vi "Noise Generation.vi"() -> ()   [LabVIEW 2019]
doc: "Generates a monotone signal. If you are setting up a demo system of active noise control, you can use this VI to simulate a noisy environment with monotone noise."
uses:
  <vilib>/sound2/lvsound2.llb/Sampling Mode.ctl
  <vilib>/sound2/lvsound2.llb/Sound Data Format.ctl
  <vilib>/sound2/lvsound2.llb/Sound Output Set Volume (Single).vi
  <vilib>/sound2/lvsound2.llb/Sound Output Write (DBL).vi
  <vilib>/measure/NI_MABase.lvlib
panel:
  in  "Amplitude":dbl(slide)=1.0 scale=0.0..1.0
  in  "Frequency (Hz)":dbl(slide)=120.0 min=50.0 max=500.0 step=1.0 scale=100.0..400.0
  in  "Stop":bool
  # "Monotone Noise Generation"
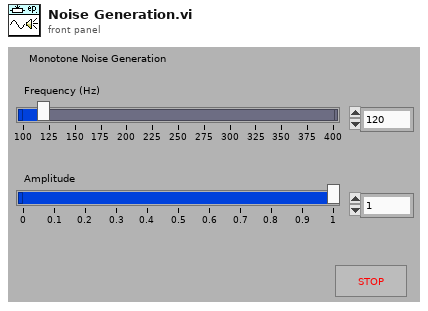
[diagram p1: front panel]
types:
  T1 = typedef "Sound Data Format.ctl" = cluster{"sample rate (S/s)":dbl, "number of channels":i32, "bits per sample":i32}
  T2 = typedef "Sampling Mode.ctl" = i32
  T3 = typedef "Sound Output Task ID.ctl" = u32
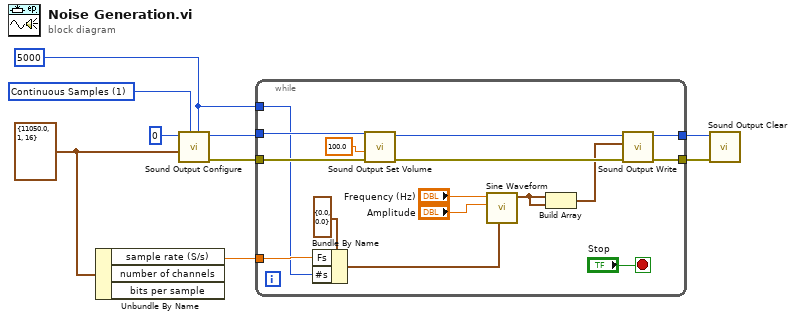
[diagram p0: block diagram]
diagram:
  w4 = T1 {"sample rate (S/s)"=11050.0, "number of channels"=1, "bits per sample"=16} ("sound format")
  w2 = 5000 ("number of samples/ch")
  w1 = T2 1 items=["Finite Samples", "Continuous Samples"] ("sample mode")
  n1 = Unbundle By Name(w4) -> ("sample rate (S/s)"=w3:dbl)  [unwired: 2 out]
  n2 = call <vilib>:"Sound Output Configure.vi"("number of samples/ch"=w2, "sample mode"=w1, "sound format"=w4, "device ID"=u32 0) -> ("error out"=w6:errorcluster, "task ID"=w8:T3)  [unwired: 1 in, 5 out]
  n3 = while {
    tunnel: w3 -> [w16]
    tunnel: w2 -> [w15]
    tunnel: w8 -> [w24]
    tunnel: [w22] -> w7
    tunnel: w6 -> [w21]
    tunnel: [w18] -> w5
    stop <- "Stop" stop-if-true
    n4 = Bundle By Name(cluster=cluster{"Fs":dbl, "#s":dbl} {"Fs"=0.0, "#s"=0.0} ("sampling info"), "Fs"=w16, "#s"=w15) -> (w12:cluster{"Fs":dbl, "#s":dbl})
    n5 = call-poly <vilib>:"Sound Output Set Volume.vi"("error in (no error)"=w21, "volume"=100.0, "task ID"=w24) -> ("error out"=w20:errorcluster, "task ID out"=w23:T3)  [unwired: 7 out]
    n6 = call <vilib>:"Sine Waveform.vi"("sampling info"=w12, "amplitude"="Amplitude", "frequency"="Frequency (Hz)") -> ("signal out"=w11:waveform(dbl))  [unwired: 4 in, 4 out]
    n7 = Build Array(w11, w11) -> (w13:waveform(dbl)[])
    n8 = call-poly <vilib>:"Sound Output Write.vi"("error in (no error)"=w20, "data"=w13, "task ID"=w23) -> ("error out"=w18:errorcluster, "task ID out"=w22:T3)  [unwired: 1 in, 6 out]
  }
  n9 = call <vilib>:"Sound Output Clear.vi"("error in (no error)"=w5, "task ID"=w7) -> ()  [unwired: 10 out]
